vi "TEST_ASIC_MAJ_(3RD).vi"(4 "Voltages comprobation":dbl[](array[numeric])=[0.05, 0.1, 0.2, 0.5, 0.8], 7 "Serial number":string="SN_023", 8 "error in":errorcluster, 9 "Cycles Burst":i32=10000, 10 "Channels":i32[](array[numeric])=[0, 1, 2, 3, 4, 5, 6], 11 "Instrument VISA in":T1={"AWG VISA"="generadorpulsos", "Oscilloscope  VISA "="Oscilloscope", "Integration Board IP"="172.16.7.43", "connection ID"=refnum, "report out"=refnum, "report file path"=path "C:/Documents and Settings/CTA_LAB01/Desktop/L0_Asic/L0 Asic Test Data"}) -> (0 "error out":errorcluster={"status"=TRUE, "code"=1, "source"="TCP Write in send_receive(SubVI).vi->sendCommand.vi->spi_control.vi->channel_conf_ASIC.vi->Disable_all_channels_ASIC.vi->TEST_ASIC_MAJ_(3RD).vi->TEST_ASIC_COMPLETE_(ALL).vi"}, 3 "Instrument VISA out":T1={"AWG VISA"="", "Oscilloscope  VISA "="", "Integration Board IP"="172.16.7.43", "connection ID"=refnum, "report out"=refnum, "report file path"=path "C:/Documents and Settings/CTA_LAB01/Desktop/L0_Asic/L0 Asic Test Data"}, 5 "Array":i32[][](array[numeric])=[[600, 502, 502, 502, 502, 502, 502], [696, 502, 502, 502, 502, 502, 502], [696, 502, 502, 502, 502, 502, 502], [696, 502, 502, 502, 502, 502, 502], [696, 502, 502, 502, 502, 502, 502]])   [LabVIEW 2009]
uses:
  <vilib>/Utility/NIReport.llb/NI_report.lvclass
  <vilib>/Utility/NIReport.llb/HTML/NI_HTML.lvclass
  <instrlib>/Agilent 81150/Agilent 81150.lvlib
  <instrlib>/Agilent 8000 Series/Agilent 8000 Series.lvlib
  <vilib>/Analysis/NI_AALBase.lvlib
panel:
  in  "Attenuation":i32[](array[numeric])=[0]
  out "Threshold array":i32[](array[numeric])=[506, 507, 508, 509, 510, 511, 512, 513, 514, 515, 516, 517, 518]
  out "read buffer 4":string="-1.181E-08;2.24E-09;9.99999E+37;2.78E-09;4.72E-02;4.90E-02\n"
  out "report file path":path=path "C:/Documents and Settings/CTA_LAB01/Desktop/L0_Asic/L0 Asic Test Data"
  in  "time to wait":dbl=10.0
  in  "Init values ch":i32[](array[numeric])=[500, 500, 500, 499, 500, 500, 500]
  out "Data output":dbl[][](array[numeric])=[[0.05, 0.0, 0.0, 500.0, 0.0, 1.999998e+38, 0.0, 3.409e-08, 0.0, 9.99999e+37, 0.0, 2.15e-09, 0.0, -1.427e-08, 0.0, 0.0, 0.16, 0.0, 500.0], [0.05, 0.0, 0.0, 501.0, 0.0, 9.99999e+37, 0.0, 9.99999e+37, 0.0, 9.99999e+37, 0.0, 2.37e-09, 0.0, -1.704e-08, 0.0, 0.0, 0.16, 0.0, 500.0], [0.05, 0.0, 0.0, 502.0, 0.0, 0.038599999999999995, 0.0, 9.99999e+37, 0.0, 9.99999e+37, 0.0, 2.27e-09, 0.0, -1.678e-08, 0.0, 0.0, 0.16, 0.0, 500.0], [0.05, 0.0, 0.0, 503.0, 0.0, 0.0503, 0.0, 9.99999e+37, 0.0, 9.99999e+37, 0.0, 2.24e-09, 0.0, -1.686e-08, 0.0, 0.0, 0.16, 0.0, 500.0], [0.05, 0.0, 0.0, 504.0, 0.0, 0.081, 0.0, 9.99999e+37, 0.0, 9.99999e+37, 0.0, 2.12e-09, 0.0, -1.736e-08, 0.0, 0.0, 0.16, 0.0, 500.0], [0.05, 0.0, 0.0, 505.0, 0.0, 0.0824, 0.0, 6.74e-09, 0.0, 9.99999e+37, 0.0, 2.16e-09, 0.0, -8.42e-09, 0.0, 0.0, 0.16, 0.0, 500.0], [0.05, 0.0, 0.0, 506.0, 0.0, 0.1013, 0.0, 4.84e-09, 0.0, 9.99999e+37, 0.0, 2.12e-09, 0.0, -1.037e-08, 0.0, 0.0, 0.16, 0.0, 500.0], [0.05, 0.0, 0.0, 507.0, 0.0, 0.1038, 0.0, 4.19e-09, 0.0, 9.99999e+37, 0.0, 2.12e-09, 0.0, -1.093e-08, 0.0, 0.0, 0.16, 0.0, 500.0], [0.05, 0.0, 0.0, 508.0, 0.0, 0.1008, 0.0, 4.09e-09, 0.0, 9.99999e+37, 0.0, 2.31e-09, 0.0, -1.064e-08, 0.0, 0.0, 0.16, 0.0, 500.0], [0.05, 0.0, 0.0, 509.0, 0.0, 0.1056, 0.0, 3.69e-09, 0.0, 9.99999e+37, 0.0, 2.12e-09, 0.0, -1.137e-08, 0.0, 0.0, 0.16, 0.0, 500.0], [0.05, 0.0, 0.0, 510.0, 0.0, 0.1066, 0.0, 3.28e-09, 0.0, 9.99999e+37, 0.0, 2.16e-09, 0.0, -1.162e-08, 0.0, 0.0, 0.16, 0.0, 500.0], [0.05, 0.0, 0.0, 511.0, 0.0, 0.10650000000000001, 0.0, 3.23e-09, 0.0, 9.99999e+37, 0.0, 2.13e-09, 0.0, -1.162e-08, 0.0, 0.0, 0.16, 0.0, 500.0], [0.05, 0.0, 0.0, 512.0, 0.0, 0.1059, 0.0, 3.01e-09, 0.0, 9.99999e+37, 0.0, 2.22e-09, 0.0, -1.163e-08, 0.0, 0.0, 0.16, 0.0, 500.0], [0.05, 0.0, 0.0, 513.0, 0.0, 0.1062, 0.0, 3.03e-09, 0.0, 9.99999e+37, 0.0, 2.12e-09, 0.0, -1.172e-08, 0.0, 0.0, 0.16, 0.0, 500.0], [0.05, 0.0, 0.0, 514.0, 0.0, 0.1052, 0.0, 2.91e-09, 0.0, 9.99999e+37, 0.0, 2.23e-09, 0.0, -1.171e-08, 0.0, 0.0, 0.16, 0.0, 500.0], [0.05, 0.0, 0.0, 515.0, 0.0, 0.1059, 0.0, 2.83e-09, 0.0, 9.99999e+37, 0.0, 2.27e-09, 0.0, -1.18e-08, 0.0, 0.0, 0.16, 0.0, 500.0], [0.05, 0.0, 0.0, 516.0, 0.0, 0.1062, 0.0, 2.76e-09, 0.0, 9.99999e+37, 0.0, 2.16e-09, 0.0, -1.193e-08, 0.0, 0.0, 0.16, 0.0, 500.0], [0.05, 0.0, 0.0, 517.0, 0.0, 0.1036, 0.0, 2.66e-09, 0.0, 9.99999e+37, 0.0, 2.12e-09, 0.0, -1.209e-08, 0.0, 0.0, 0.16, 0.0, 500.0], [0.05, 0.0, 0.0, 518.0, 0.0, 0.09620000000000001, 0.0, 2.78e-09, 0.0, 9.99999e+37, 0.0, 2.24e-09, 0.0, -1.181e-08, 0.0, 0.0, 0.16, 0.0, 500.0]]
  out "time for inner bucle":u32=225
  out "read buffer 3":string
  out "appended array":dbl[](array[numeric])=[0.09620000000000001, 0.0, 2.78e-09, 0.0, 9.99999e+37, 0.0, 2.24e-09, 0.0, -1.181e-08, 0.0, 0.0]
  out "points quantity":dbl
  out "Numeric":i32=240563532
  in  "Save NOW!":bool
  in  "End 2":bool
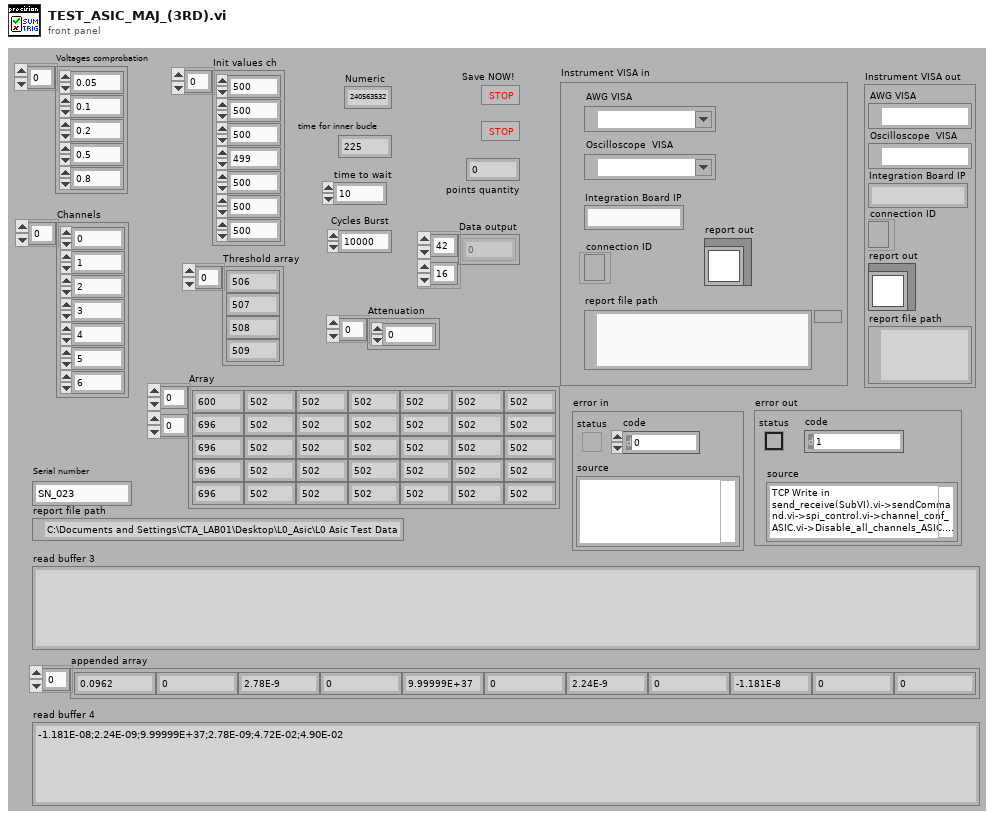
[diagram p1: front panel]
types:
  T1 = cluster{"AWG VISA":refnum<visa-resource-name>, "Oscilloscope  VISA ":refnum<visa-resource-name>, "Integration Board IP":string, "connection ID":refnum<k5>, "report out":refnum<class "NI_report.lvclass">, "report file path":path}
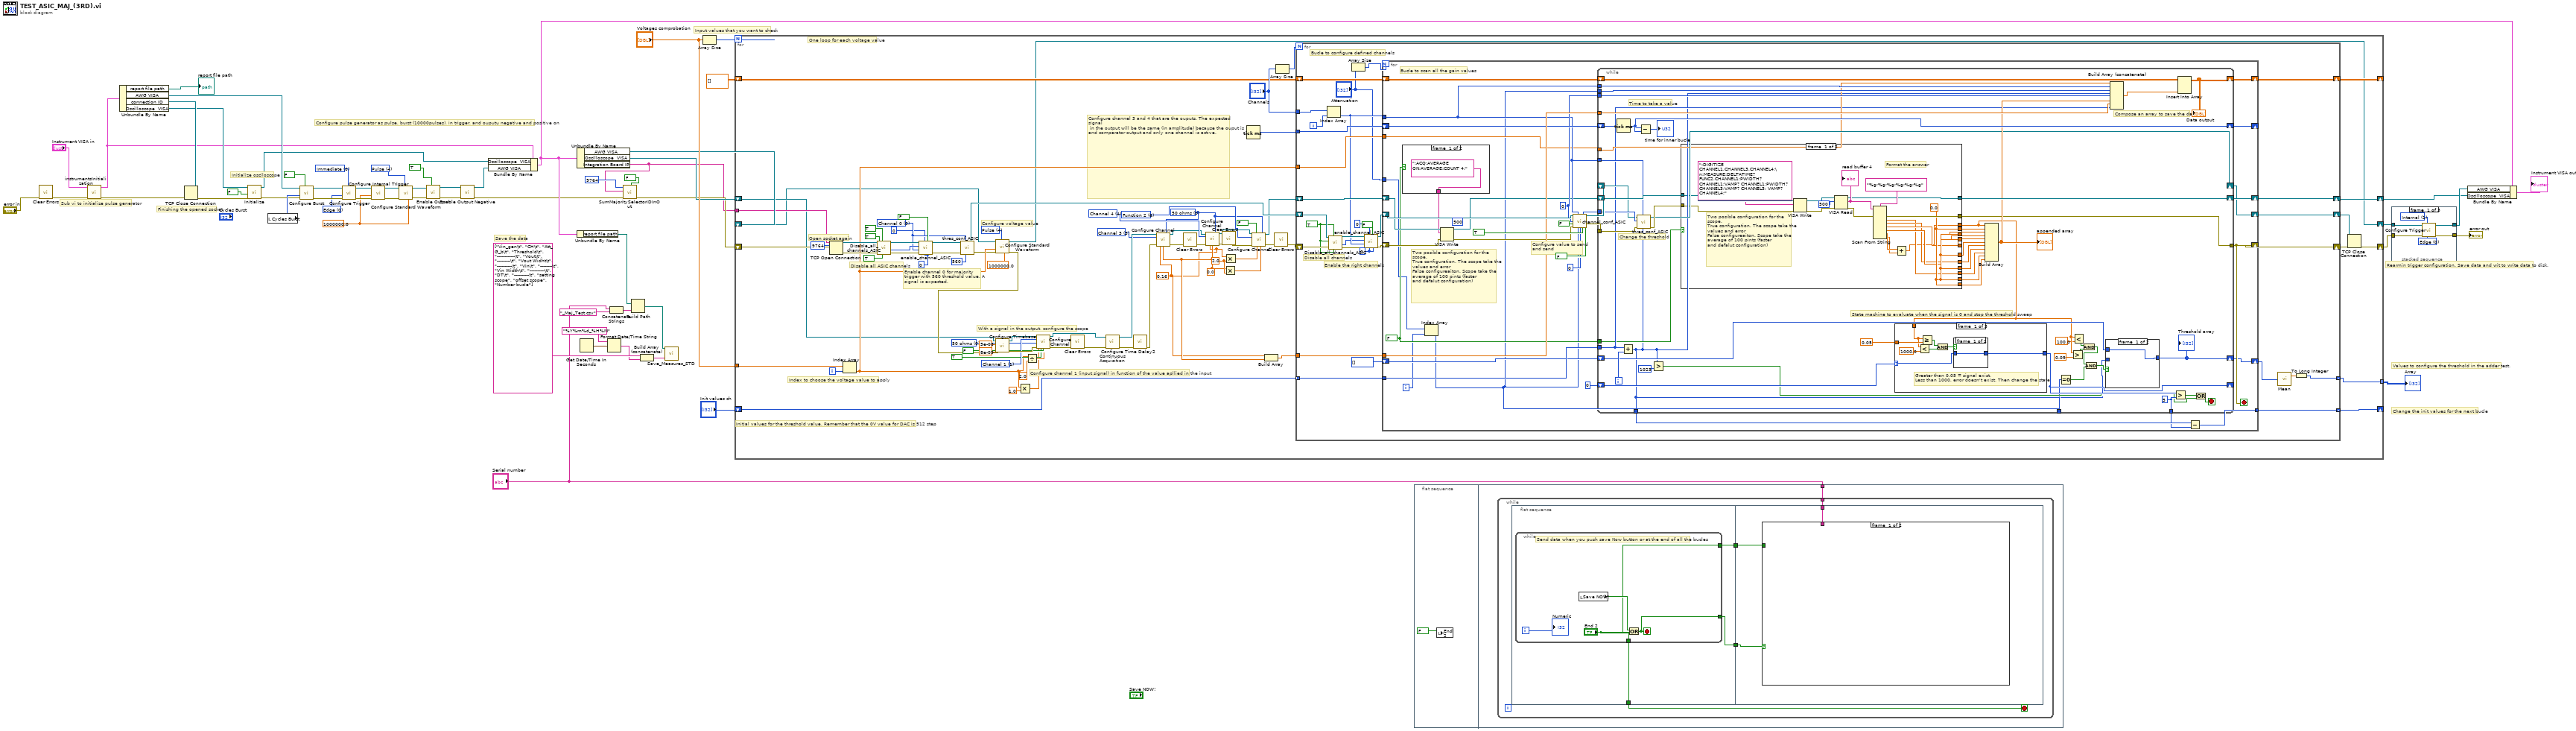
[diagram p0: block diagram]
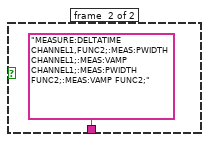
[diagram p2: hidden frame]
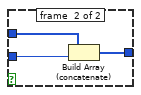
[diagram p3: hidden frame]
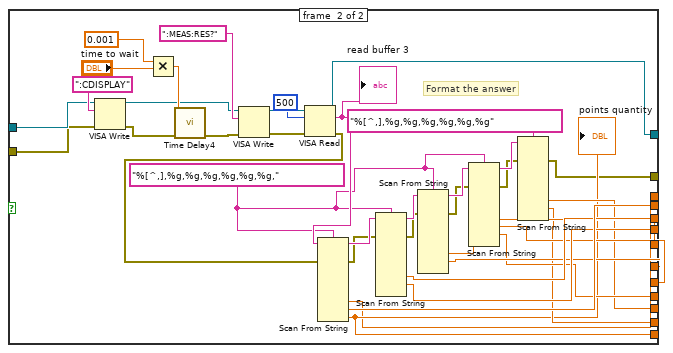
[diagram p4: hidden frame]
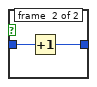
[diagram p5: hidden frame]
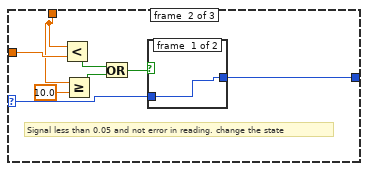
[diagram p6: hidden frame]
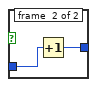
[diagram p7: hidden frame]
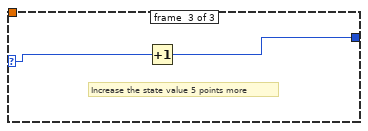
[diagram p8: hidden frame]
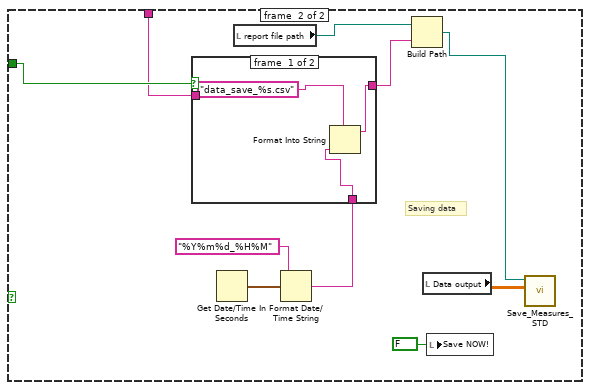
[diagram p9: hidden frame]
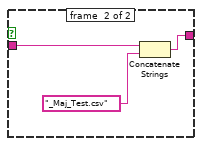
[diagram p10: hidden frame]
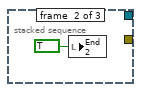
[diagram p11: hidden frame]
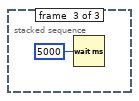
[diagram p12: hidden frame]
diagram:
  w25 = 1000000.0 ("Frequency (1000.0 Hz)")
  w51 = u16 0 items=["Immediate", "Internal", "External", "Software Trigger Function"] ("Trigger Source (0: Immediate)")
  w52 = u16 0 items=["Edge", "Level"] ("Trigger Mode (0: Edge)")
  w56 = u16 4 items=["Sine", "Square", "Ramp Up", "Ramp Down", "Pulse", "Noise", "DC"] ("Waveform (0: Sine)")
  # "Save the data"
  # "Values to configure the threshold in the adder test."
  # "Rearmin trigger configuration. Save data and wit to write data to disk."
  # "Change the init values for the next bucle"
  # "Input values that you want to check"
  # "Configure pulse generator as pulse, burst (10000pulses), in trigger, and ouputu negative and positive on"
  # "Initialize osciloscope"
  # "Finishing the opened socket"
  # "Sub vi to initialize pulse generator"
  n1 = call <vilib>:"Clear Errors.vi"("error in (no error)"="error in") -> ("error out"=w58:errorcluster)  [unwired: 6 in]
  n2 = call "instrumentsInitialization.vi"("error in"=w58, "Instrument VISA in"="Instrument VISA in") -> ("error out"=w45:errorcluster, "Instrument VISA out"=w36:T1)  [unwired: 8 in]
  n3 = Unbundle By Name(w36) -> ("report file path"=→"report file path":path, "AWG VISA"=w41:refnum<visa-resource-name>, "connection ID"=w46:refnum<k5>, "Oscilloscope  VISA"=w42:refnum<visa-resource-name>)
  n4 = TCP Close Connection(connection ID=w46, error in (no error)=w45) -> (error out=w40:errorcluster)  [unwired: 1 in, 1 out]
  n5 = call <instrlib>:"Initialize.vi"("error in (no error)"=w40, "Reset (True)"=FALSE ("ID Query (True)"), "VISA resource name"=w42) -> ("error out"=w21:errorcluster, "VISA resource name out"=w39:refnum<visa-resource-name>)  [unwired: 7 in]
  n6 = local read "Cycles Burst"() -> (w55:i32)
  n7 = call <instrlib>:"Configure Burst.vi"("Enable Burst (F: Disable)"=FALSE, "error in (no error)"=w21, "Burst Count (2)"=w55, "VISA resource name"=w41) -> ("error out"=w54:errorcluster, "VISA resource name out"=w53:refnum<visa-resource-name>)  [unwired: 6 in]
  n8 = call <instrlib>:"Configure Trigger.vi"("Trigger Source (0: Immediate)"=w51, "error in (no error)"=w54, "Trigger Mode (0: Edge)"=w52, "VISA resource name"=w53) -> ("error out"=w50:errorcluster, "VISA resource name out"=w49:refnum<visa-resource-name>)  [unwired: 6 in]
  n9 = call <instrlib>:"Configure Internal Trigger.vi"("error in (no error)"=w50, "Frequency (100000.0 Hz)"=w25, "VISA resource name"=w49) -> ("error out"=w47:errorcluster, "VISA resource name out"=w48:refnum<visa-resource-name>)  [unwired: 7 in]
  n10 = call <instrlib>:"Configure Standard Waveform.vi"("Frequency (1000.0 Hz)"=w25, "Waveform (0: Sine)"=w56, "error in (no error)"=w47, "VISA resource name"=w48) -> ("error out"=w38:errorcluster, "VISA resource name out"=w37:refnum<visa-resource-name>)  [unwired: 6 in]
  n11 = call <instrlib>:"Enable Output.vi"("Enable Output (T: Enable)"=TRUE, "error in (no error)"=w38, "VISA resource name"=w37) -> ("error out"=w24:errorcluster, "VISA resource name out"=w23:refnum<visa-resource-name>)  [unwired: 7 in]
  n12 = call <instrlib>:"Enable Output Negative.vi"("error in (no error)"=w24, "VISA resource name"=w23) -> ("error out"=w4:errorcluster, "VISA resource name out"=w22:refnum<visa-resource-name>)  [unwired: 8 in]
  n13 = Bundle By Name(cluster=w36, "Oscilloscope  VISA"=w39, "AWG VISA"=w22) -> (w7:T1)
  n14 = Unbundle By Name(w7) -> ("report file path"=w8:path)
  n15 = Unbundle By Name(w7) -> ("AWG VISA"=w19:refnum<visa-resource-name>, "Oscilloscope  VISA"=w20:refnum<visa-resource-name>, "Integration Board IP"=w2:string)
  n16 = Get Date/Time In Seconds() -> (seconds since 1Jan1904=w13:timestamp)
  n17 = Format Date/Time String(time format string (%c)="%Y%m%d_%H%M", seconds (now)=w13) -> (date/time string=w11:string)  [unwired: 1 in]
  n18 = Concatenate Strings("Serial number", "_Maj_Test.csv" ("format string")) -> (w9:string)
  n19 = call "SumMajoritySelectorIDInOut.vi"("On Sum\nOff Majority"=FALSE, "error in (no error)"=w4, "address"=w2, "remote port or service name"=u16 9764) -> ("error out"=w5:errorcluster)  [unwired: 7 in]
  n20 = Build Path(base path=w8, name or relative path=w9) -> (appended path=w16:path)
  n21 = Build Array (concatenate)(string[] ["Vin_gen\t", "CH\t", "Att_G_b\t", "Threshold\t", "------------\t", "Vout\t", "---------\t", "Vout Widht\t", "----------\t", "Vin\t", "--------\t", "Vin Width\t", "----------\t", "DT\t", "----------\t", "setting scope", "offset scope", "Number bucle"] ("appended array"), w11) -> (w14:string[])
  n22 = call "Save_Measures_STD.vi"("appended array"=w14, "file path (dialog if empty)"=w16) -> ()  [unwired: 10 in]
  n23 = Array Size(array="Voltages comprobation") -> (size(s)=w30:i32)
  n24 = for {
    N: w30 -> [_]
    tunnel: w2 -> [w138]
    tunnel: "Voltages comprobation" -> [w137]
    shift-right: [w97] -> _
    shift-left: dbl[][] [] -> [w98]
    shift-right: [w95] -> _
    shift-left: "Init values ch" -> [w96]
    shift-right: [w73] -> w27
    shift-left: w20 -> [w69]
    shift-right: [w139] -> w33
    shift-left: w5 -> [w70]
    shift-right: [w68] -> w26
    shift-left: w19 -> [w62]
    tunnel: [w61] -> w17 mode=indexing
    i -> [w93]
    w74 = 0.16 ("Vertical Range (2.0 V)")
    w75 = 0.0 ("Vertical Offset (0.0 V)")
    w92 = u32 0 ("Clip_sel_b")
    w105 = 2.0 ("y")
    w77 = u32 0 items=["50 ohms", "1 Mohms"] ("Input Impedance (1: 1 Mohms)")
    w85 = u16 0 items=["Channel 0", "Channel 1", "Channel 2", "Channel 3", "Channel 4", "Channel 5", "Channel 6"] ("Channel")
    w125 = u32 0 items=["50 ohms", "1 Mohms"] ("Input Impedance (1: 1 Mohms)")
    w128 = 1 items=["Channel 1"=1, "Channel 2"=2, "Channel 3"=3, "Channel 4"=4] ("Channel (1: Channel 1)")
    w109 = u16 6 items=["Function 1"=5, "Function 2"=6, "Function 3"=7, "Function 4"=8] ("Math Channel (5: Function 1)")
    w76 = 3 items=["Channel 1"=1, "Channel 2"=2, "Channel 3"=3, "Channel 4"=4] ("Channel (1: Channel 1)")
    w123 = 4 items=["Channel 1"=1, "Channel 2"=2, "Channel 3"=3, "Channel 4"=4] ("Channel (1: Channel 1)")
    w135 = u16 4 items=["Sine", "Square", "Ramp Up", "Ramp Down", "Pulse", "Noise", "DC"] ("Waveform (0: Sine)")
    # "Initial values for the threshold value. Remember that the 0V value for DAC is 512 step"
    # "Configure channel 3 and 4 that are the ouputs. The expected signal\n in the output will be the same (in amplitude) because the ouput is and comparator output and only one channel is active."
    # "Configure channel 1 (input signal) in function of the value apllied in the input"
    # "With a signal in the output, configure the scope"
    # "Enable channel 0 for majority trigger with 560 threshold value. A signal is expected."
    # "Disable all ASIC channels"
    # "Open socket again"
    # "Configure voltage value"
    # "Index to choose the voltage value to apply"
    # "One loop for each voltage value"
    n25 = TCP Open Connection(address=w138, remote port or service name=u16 9764, error in (no error)=w70) -> (connection ID=w119:refnum<k5>, error out=w118:errorcluster)  [unwired: 2 in]
    n26 = Index Array(array=w137, index=w93) -> (element=w94:dbl)
    n27 = call "Disable_all_channels_ASIC.vi"("CompBuf_en_b"=TRUE, "Att_en_b"=TRUE, "error in"=w118, "Clip_en_b"=TRUE, "connection ID"=w119) -> ("error out"=w117:errorcluster, "id_out"=w115:i32, "connection ID out"=w116:refnum<k5>)  [unwired: 4 in]
    n28 = call "enable_channel_ASIC.vi"("Clip_sel_b"=w92, "maj/sum"=FALSE, "Ib_clipVb"=w92, "Att gain"=u32 0, "error in"=w117, "Channel"=w85, "id_in"=w115, "connection ID"=w116) -> ("error out"=w88:errorcluster, "connection ID out"=w90:refnum<k5>)  [unwired: 1 in, 1 out]
    n29 = call "thres_conf_ASIC.vi"("threshold"=u32 560, "Ring"=w85, "error out 3"=w88, "connection ID"=w90) -> ("error out 2"=w87:errorcluster, "connection ID out"=w89:refnum<k5>)  [unwired: 4 in, 2 out]
    n30 = call <instrlib>:"Configure Standard Waveform.vi"("Frequency (1000.0 Hz)"=1000000.0, "Waveform (0: Sine)"=w135, "error in (no error)"=w87, "Amplitude (1.0 Vpp)"=w94, "VISA resource name"=w62) -> ("error out"=w132:errorcluster, "VISA resource name out"=w68:refnum<visa-resource-name>)  [unwired: 5 in]
    n31 = call <instrlib>:"Configure Timebase.vi"("error in (no error)"=w132, "Position (0.0 s)"=8e-09, "Timebase (0.005 s)"=5e-08, "VISA resource name"=w69) -> ("error out"=w129:errorcluster, "VISA resource name out"=w130:refnum<visa-resource-name>)  [unwired: 6 in]
    n32 = Multiply(x=w94, y=1.0) -> (x*y=w106:dbl)
    n33 = Divide(x=w94, y=2.0) -> (x/y=w114:dbl)
    n34 = call <instrlib>:"Configure Channel.vi"("VISA resource name"=w130, "Enable Channel (Enable)"=TRUE, "BW Limit 20MHz (Disable)"=FALSE, "Input Impedance (1: 1 Mohms)"=w125, "Channel (1: Channel 1)"=w128, "error in (no error)"=w129, "Vertical Range (2.0 V)"=w106, "Vertical Offset (0.0 V)"=w114) -> ("VISA resource name out"=w65:refnum<visa-resource-name>, "error out"=w127:errorcluster)  [unwired: 6 in]
    n35 = call <vilib>:"Clear Errors.vi"("error in (no error)"=w127) -> ("error out"=w64:errorcluster)  [unwired: 6 in]
    n36 = call <instrlib>:"Configure Continuous Acquisition.vi"("error in (no error)"=w64, "VISA resource name"=w65) -> ("error out"=w108:errorcluster, "VISA resource name out"=w78:refnum<visa-resource-name>)  [unwired: 8 in]
    n37 = call "Time Delay2"("error in (no error)"=w108) -> ("error out"=w79:errorcluster)  [unwired: 10 in]
    n38 = call <instrlib>:"Configure Channel.vi"("VISA resource name"=w78, "Input Impedance (1: 1 Mohms)"=w77, "Channel (1: Channel 1)"=w76, "error in (no error)"=w79, "Vertical Range (2.0 V)"=w74, "Vertical Offset (0.0 V)"=w75) -> ("VISA resource name out"=w80:refnum<visa-resource-name>, "error out"=w81:errorcluster)  [unwired: 8 in]
    n39 = call <vilib>:"Clear Errors.vi"("error in (no error)"=w81) -> ("error out"=w120:errorcluster)  [unwired: 6 in]
    n40 = call <instrlib>:"Configure Channel.vi"("VISA resource name"=w80, "Input Impedance (1: 1 Mohms)"=w77, "Channel (1: Channel 1)"=w123, "error in (no error)"=w120, "Vertical Range (2.0 V)"=w74, "Vertical Offset (0.0 V)"=w75) -> ("VISA resource name out"=w111:refnum<visa-resource-name>, "error out"=w121:errorcluster)  [unwired: 8 in]
    n41 = call <vilib>:"Clear Errors.vi"("error in (no error)"=w121) -> ("error out"=w112:errorcluster)  [unwired: 6 in]
    n42 = Multiply(x=w75, y=w105) -> (x*y=w104:dbl)
    n43 = Multiply(x=w74, y=w105) -> (x*y=w110:dbl)
    n44 = Tick Count (ms)() -> (millisecond timer value=w102:u32)
    n45 = call <instrlib>:"Configure Channel.vi"("VISA resource name"=w111, "Enable Channel (Enable)"=FALSE, "Input Impedance (1: 1 Mohms)"=w77, "Channel (1: Channel 1)"=w109, "error in (no error)"=w112, "Vertical Range (2.0 V)"=w110, "Vertical Offset (0.0 V)"=w104) -> ("VISA resource name out"=w72:refnum<visa-resource-name>, "error out"=w113:errorcluster)  [unwired: 7 in]
    n46 = Build Array(w74, w75) -> (w101:dbl[])
    n47 = call <vilib>:"Clear Errors.vi"("error in (no error)"=w113) -> ("error out"=w103:errorcluster)  [unwired: 6 in]
    n48 = Array Size(array="Channels") -> (size(s)=w100:i32)
    n49 = for {
      N: w100 -> [_]
      tunnel: w102 -> [w169]
      tunnel: w101 -> [w168]
      tunnel: "Channels" -> [w167]
      shift-right: [w170] -> w97
      shift-left: w98 -> [w165]
      tunnel: w96 -> [w164] mode=indexing
      tunnel: [w163] -> w95 mode=indexing
      tunnel: w94 -> [w162]
      shift-right: [w161] -> w73
      shift-left: w72 -> [w160]
      shift-right: [w159] -> w71
      shift-left: w103 -> [w156]
      shift-right: [w158] -> w67
      shift-left: w89 -> [w153]
      tunnel: [w142] -> w61 mode=indexing
      i -> [w166]
      w150 = u32 0 ("Ib_clipVb")
      w151 = TRUE ("Att_en_b")
      # "Enable the right channels"
      # "Disable all channels"
      # "Bucle to configure defined channels"
      n50 = Index Array(array=w167, index=w166) -> (element=w148:i32)
      n51 = call "Disable_all_channels_ASIC.vi"("CompBuf_en_b"=w151, "Att_en_b"=w151, "error in"=w156, "Clip_en_b"=w151, "connection ID"=w153) -> ("error out"=w157:errorcluster, "id_out"=w147:i32, "connection ID out"=w154:refnum<k5>)  [unwired: 4 in]
      n52 = Array Size(array="Attenuation") -> (size(s)=w141:i32)
      n53 = call "enable_channel_ASIC.vi"("Clip_sel_b"=w150, "maj/sum"=FALSE, "Ib_clipVb"=w150, "Att gain"=u32 0, "error in"=w157, "Channel"=w148, "id_in"=w147, "connection ID"=w154) -> ("error out"=w155:errorcluster, "connection ID out"=w152:refnum<k5>)  [unwired: 1 in, 1 out]
      n54 = for {
        N: w141 -> [_]
        shift-right: [w197] -> w159
        shift-left: w155 -> [w182]
        shift-right: [w198] -> w170
        shift-left: w165 -> [w205]
        shift-right: [w199] -> w161
        shift-left: w160 -> [w181]
        shift-right: [w191] -> w158
        shift-left: w152 -> [w204]
        tunnel: w168 -> [w202]
        shift-right: [w200] -> _
        shift-left: w169 -> [w201]
        tunnel: w148 -> [w190]
        tunnel: w164 -> [w188]
        tunnel: [w183] -> w163
        tunnel: w162 -> [w186]
        shift-right: [w175] -> w143
        shift-left: i32[] [] -> [w174]
        tunnel: "Attenuation" -> [w173]
        i -> [w172]
        stop <- w197 stop-if-true
        w176 = FALSE
        (unwired) u32 500 ("byte count")
        w192 = u32 0 ("Ib_ClipVb")
        # "Configure value to send and send"
        # "Two posible configuration for the scope. \nTrue configuration. The scope take the values and error\nFalse configureaiton. Scope take the average of 100 pints (faster\nand defalut configuration)"
        # "Bucle to scan all the gain values"
        n55 = case shown="False" w176 {
          tunnel: [":ACQ:AVERAGE ON;AVERAGE:COUNT 4;" ("write buffer") "MEASURE:DELTATIME CHANNEL1,FUNC2;:MEAS:PWIDTH CHANNEL1;:MEAS:VAMP CHANNEL1;:MEAS:PWIDTH FUNC2;:MEAS:VAMP FUNC2;" ("write buffer")] -> w180
          frame #0 {
          }
          frame #1 {
          }
        }
        n56 = Index Array(array=w173, index=w172) -> (element=w171:i32)
        n57 = VISA Write(VISA resource name=w181, write buffer=w180, error in (no error)=w182) -> (VISA resource name out=w178:refnum<visa-resource-name>, error out=w177:errorcluster)  [unwired: 1 out]
        n58 = call "channel_conf_ASIC.vi"("connection ID"=w204, "Ring"=w190, "Clip_sel_b"=w192, "CompBuf_en_b"=FALSE, "error out"=w177, "Att gain"=w171, "Ib_ClipVb"=u32 0, "Clip_en_b"=TRUE, "Att_en_b"=FALSE) -> ("Id out"=w189:i32, "connection ID out"=w179:refnum<k5>, "error out 2"=w194:errorcluster)  [unwired: 2 in, 2 out]
        n59 = while {
          tunnel: w202 -> [w259]
          tunnel: [w242] -> w197
          tunnel: w194 -> [w236]
          tunnel: w192 -> [w240]
          tunnel: w190 -> [w239]
          tunnel: w171 -> [w238]
          tunnel: w190 -> [w234]
          tunnel: w189 -> [w233]
          tunnel: w188 -> [w221]
          shift-right: [w228] -> _
          shift-left: 0 -> [w231]
          tunnel: [w208] -> w185
          tunnel: w186 -> [w229]
          tunnel: [w227] -> w184
          shift-right: [w257] -> w200
          shift-left: w201 -> [w258]
          shift-right: [w255] -> w199
          shift-left: w178 -> [w241]
          shift-right: [w235] -> w191
          shift-left: w179 -> [w226]
          shift-right: [w252] -> w198
          shift-left: w205 -> [w260]
          tunnel: w176 -> [w220]
          shift-right: [w218] -> w175
          shift-left: w174 -> [w217]
          tunnel: w171 -> [w214]
          i -> [w232]
          stop <- w223 stop-if-true
          w227 = 5 ("y")
          # "State machine to evaluate when the signal is 0 and stop the threshold sweep"
          # "Compose an array to save the data"
          # "Change the threshold"
          # "Time to take a value"
          n60 = Tick Count (ms)() -> (millisecond timer value=w257:u32)
          n61 = Add(x=w221, y=w232) -> (x+y=w208:i32)
          n62 = call "thres_conf_ASIC.vi"("threshold"=w208, "Ring"=w234, "error out 3"=w236, "Id in"=w233, "connection ID"=w226) -> ("error out 2"=w237:errorcluster, "connection ID out"=w235:refnum<k5>)  [unwired: 3 in, 2 out]
          n63 = Subtract(x=w257, y=w258) -> (x-y=→"time for inner bucle":u32)
          n64 = Greater?(x=w208, y=1023) -> (0:w222:bool)
          n65 = case shown="False" w220 {
            tunnel: [w279 w313] -> w255
            tunnel: [w277 w312] -> w254
            tunnel: [w273 w305] -> w251
            tunnel: [w277 w304] -> w250
            tunnel: [w274 w303] -> w249
            tunnel: [w277 w302] -> w248
            tunnel: [w272 w301] -> w247
            tunnel: [w277 w300] -> w246
            tunnel: [w271 w299] -> w245
            tunnel: [w277 w298] -> w244
            tunnel: [w277 w297] -> w243
            tunnel: [w278 w295] -> w242
            tunnel: w241 -> [w280 w288]
            tunnel: w237 -> [w269 w286]
            tunnel: [w266 w285] -> w213
            frame #0 {
              w277 = 0.0 ("points quantity")
              # "Format the answer"
              # "Two posible configuration for the scope. \nTrue configuration. The scope take the values and error\nFalse configureaiton. Scope take the average of 100 pints (faster\nand defalut configuration)"
              n66 = VISA Write(VISA resource name=w280, write buffer=":DIGITIZE CHANNEL1,CHANNEL3,CHANNEL4;\n:MEASURE:DELTATIME? FUNC2,CHANNEL1;PWIDTH? CHANNEL1;VAMP? CHANNEL1;PWIDTH? CHANNEL3;VAMP? CHANNEL3; VAMP? CHANNEL4;", error in (no error)=w269) -> (VISA resource name out=w275:refnum<visa-resource-name>, error out=w276:errorcluster)  [unwired: 1 out]
              n67 = VISA Read(VISA resource name=w275, byte count=u32 500, error in (no error)=w276) -> (VISA resource name out=w279:refnum<visa-resource-name>, read buffer=w283:string, error out=w281:errorcluster)  [unwired: 1 out]
              "read buffer 4" <- w283
              n68 = Scan From String(format string="%g;%g;%g;%g;%g;%g", input string=w283, error in=w281) -> (error out=w278:errorcluster, output 1=w271:dbl, output 2=w272:dbl, output 3=w274:dbl, output 4=w273:dbl, output 5=w268:dbl, output 6=w267:dbl)  [unwired: 7 in, 2 out]
              n69 = Add(x=w268, y=w267) -> (x+y=w266:dbl)
            }
            frame #1 {
              w307 = "%[^,],%g,%g,%g,%g,%g,%g," ("format string")
              # "Format the answer"
              n70 = VISA Write(VISA resource name=w288, write buffer=":CDISPLAY", error in (no error)=w286) -> (VISA resource name out=w290:refnum<visa-resource-name>, error out=w287:errorcluster)  [unwired: 1 out]
              n71 = Multiply(x=0.001, y="time to wait") -> (x*y=w315:dbl)
              n72 = call "Time Delay4"("error in (no error)"=w287, "Delay Time (s)"=w315) -> ("error out"=w314:errorcluster)  [unwired: 9 in]
              n73 = VISA Write(VISA resource name=w290, write buffer=":MEAS:RES?", error in (no error)=w314) -> (VISA resource name out=w322:refnum<visa-resource-name>, error out=w321:errorcluster)  [unwired: 1 out]
              n74 = VISA Read(VISA resource name=w322, byte count=u32 500, error in (no error)=w321) -> (VISA resource name out=w313:refnum<visa-resource-name>, read buffer=w318:string, error out=w296:errorcluster)  [unwired: 1 out]
              "read buffer 3" <- w318
              n75 = Scan From String(format string=w307, input string=w318, error in=w296) -> (remaining string=w311:string, error out=w291:errorcluster, output 5=w285:dbl, output 6=w312:dbl, output 7=w297:dbl)  [unwired: 12 in, 1 out]
              "points quantity" <- w297
              n76 = Scan From String(format string=w307, input string=w311, error in=w291) -> (remaining string=w308:string, error out=w292:errorcluster, output 5=w305:dbl, output 6=w304:dbl)  [unwired: 13 in, 1 out]
              n77 = Scan From String(format string=w307, input string=w308, error in=w292) -> (remaining string=w309:string, error out=w293:errorcluster, output 5=w303:dbl, output 6=w302:dbl)  [unwired: 13 in, 1 out]
              n78 = Scan From String(format string=w307, input string=w309, error in=w293) -> (remaining string=w310:string, error out=w294:errorcluster, output 5=w301:dbl, output 6=w300:dbl)  [unwired: 13 in, 1 out]
              n79 = Scan From String(format string="%[^,],%g,%g,%g,%g,%g,%g", input string=w310, error in=w294) -> (error out=w295:errorcluster, output 5=w299:dbl, output 6=w298:dbl)  [unwired: 13 in, 2 out]
            }
          }
          n80 = case shown="1" w231 {
            selector: w231 -> [w323 w334 w345]
            tunnel: [w330 w340 w346] -> w228
            tunnel: w213 -> [w328 w335 _]
            tunnel: 0.05 ("y") -> [w329 w341 _]
            frame #0 {
              # "Greater than 0.05 = signal exist.\nLess than 1000, error doesn't exist. Then change the state"
              n81 = Less?(x=w328, y=1000.0) -> (x < y?=w324:bool)
              n82 = Greater Or Equal?(x=w328, y=w329) -> (x >= y?=w325:bool)
              n83 = And(x=w325, y=w324) -> (x .and. y?=w326:bool)
              n84 = case shown="True" w326 {
                tunnel: w323 -> [w331 w332]
                tunnel: [w331 w333] -> w330
                frame #0 {
                }
                frame #1 {
                  n85 = Increment(x=w332) -> (x+1=w333:i32)
                }
              }
            }
            frame #1 {
              # "Signal less than 0.05 and not error in reading. change the state"
              n86 = Less?(x=w335, y=w341) -> (x < y?=w338:bool)
              n87 = Greater Or Equal?(x=w335, y=10.0) -> (x >= y?=w337:bool)
              n88 = Or(x=w338, y=w337) -> (x .or. y?=w339:bool)
              n89 = case shown="False" w339 {
                tunnel: w334 -> [w342 w344]
                tunnel: [w342 w343] -> w340
                frame #0 {
                }
                frame #1 {
                  n90 = Increment(x=w344) -> (x+1=w343:i32)
                }
              }
            }
            frame #2 {
              # "Increase the state value 5 points more"
              n91 = Increment(x=w345) -> (x+1=w346:i32)
            }
          }
          n92 = Build Array(w213, w254, w251, w250, w249, w248, w247, w246, w245, w244, w243) -> (w253:dbl[])
          "appended array" <- w253
          n93 = Equal To 0?(x=w214) -> (x = 0?=w215:bool)
          n94 = Greater?(x=w213, y=0.09) -> (0:w210:bool)
          n95 = Less?(x=w213, y=100.0) -> (x < y?=w211:bool)
          n96 = And(x=w211, y=w210) -> (x .and. y?=w209:bool)
          n97 = And(x=w209, y=w215) -> (x .and. y?=w216:bool)
          n98 = case shown="True" w216 {
            tunnel: w208 -> [_ w265]
            tunnel: w217 -> [w262 w264]
            tunnel: [w262 w263] -> w218
            frame #0 {
            }
            frame #1 {
              n99 = Build Array (concatenate)(w264, w265) -> (w263:i32[])
            }
          }
          "Threshold array" <- w218
          n100 = Build Array (concatenate)(w229, w239, w238, w208, w240, w253, w259, w221) -> (w261:dbl[])
          n101 = Greater?(x=w228, y=w227) -> (0:w224:bool)
          n102 = Insert Into Array(array=w260, new element=w261) -> (w252:dbl[][])  [unwired: 2 in]
          "Data output" <- w252
          n103 = Or(x=w224, y=w222) -> (x .or. y?=w223:bool)
        }
        n104 = Subtract(x=w185, y=w184) -> (x-y=w183:i32)
      }
      n105 = call <vilib>:"Mean.vi"("X"=w143) -> ("mean"=w144:dbl)  [unwired: 1 out]
      n106 = To Long Integer(number=w144) -> (32bit integer=w142:i32)
    }
    n107 = TCP Close Connection(connection ID=w67, error in (no error)=w71) -> (error out=w139:errorcluster)  [unwired: 1 in, 1 out]
  }
  "Array" <- w17
  n108 = flat-sequence {
    tunnel: "Serial number" -> [w348]
    frame #0 {
      n109 = local write "End 2"(FALSE ("End")) -> ()
    }
    frame #1 {
      n110 = while {
        tunnel: w348 -> [w349]
        stop <- w350 stop-if-true
        n111 = flat-sequence {
          tunnel: [w355] -> w352
          tunnel: [w354] -> w351
          tunnel: [w353] -> w350
          tunnel: w352 -> [w362]
          tunnel: w351 -> [w361]
          tunnel: w349 -> [w360]
          frame #0 {
            n112 = while {
              tunnel: [w358] -> w355
              tunnel: ["End 2"] -> w354
              tunnel: ["End 2"] -> w353
              i -> [w357]
              stop <- w358 stop-if-true
              # "Send data when you push save Now button or at the end of all the bucles"
              n113 = local read "Save NOW!"() -> (w359:bool)
              n114 = Or(x=w359, y="End 2") -> (x .or. y?=w358:bool)
              "Numeric" <- w357
            }
          }
          frame #1 {
            n115 = case shown="True" w362 {
              tunnel: w361 -> [_ w369]
              tunnel: w360 -> [_ w363]
              frame #0 {
              }
              frame #1 {
                # "Saving data"
                n116 = Get Date/Time In Seconds() -> (seconds since 1Jan1904=w367:timestamp)
                n117 = local read "report file path"() -> (w371:path)
                n118 = Format Date/Time String(time format string (%c)="%Y%m%d_%H%M", seconds (now)=w367) -> (date/time string=w365:string)  [unwired: 1 in]
                n119 = case shown="True" w369 {
                  tunnel: [w374 w378] -> w368
                  tunnel: w365 -> [w373 _]
                  tunnel: w363 -> [_ w376]
                  frame #0 {
                    n120 = Format Into String(format string="data_save_%s.csv", w373) -> (resulting string=w374:string)  [unwired: 2 in, 1 out]
                  }
                  frame #1 {
                    n121 = Concatenate Strings(w376, "_Maj_Test.csv" ("format string")) -> (w378:string)
                  }
                }
                n122 = Build Path(base path=w371, name or relative path=w368) -> (appended path=w372:path)
                n123 = local read "Data output"() -> (w364:dbl[][])
                n124 = local write "Save NOW!"(FALSE ("Save NOW!")) -> ()
                n125 = call "Save_Measures_STD.vi"("Data in"=w364, "file path (dialog if empty)"=w372) -> ()  [unwired: 10 in]
              }
            }
          }
        }
      }
    }
  }
  n126 = stacked-sequence {
    tunnel: w33 -> [w382 _ _]
    tunnel: [w381 _ _] -> w18
    tunnel: w26 -> [w380 _ _]
    tunnel: [w379 _ _] -> w28
    frame #0 {
      w383 = u16 1 items=["Immediate", "Internal", "External", "Software Trigger Function"] ("Trigger Source (0: Immediate)")
      w384 = u16 0 items=["Edge", "Level"] ("Trigger Mode (0: Edge)")
      n127 = call <instrlib>:"Configure Trigger.vi"("Trigger Source (0: Immediate)"=w383, "error in (no error)"=w382, "Trigger Mode (0: Edge)"=w384, "VISA resource name"=w380) -> ("error out"=w381:errorcluster, "VISA resource name out"=w379:refnum<visa-resource-name>)  [unwired: 6 in]
    }
    frame #1 {
      n128 = local write "End 2"(TRUE ("End 2")) -> ()
    }
    frame #2 {
      n129 = Wait (ms)(milliseconds to wait=u32 5000) -> ()  [unwired: 1 out]
    }
  }
  "error out" <- w18
  n130 = Bundle By Name(cluster=w7, "AWG VISA"=w28, "Oscilloscope  VISA"=w27) -> (→"Instrument VISA out":T1)
